vi "CryoCooler Alarm Check.vi"(8 "error in (no error)":errorcluster, 10 "Cryo Alarms":T1, 11 "Array":T3[](array[typedef])) -> (0 "error out":errorcluster, 1 "shutdown?":bool, 2 "Alarms":T2[](array[typedef]), 3 "Alarm":bool)   [LabVIEW 2024]
uses:
  Cryo Cooler/CryoCoolerAVC/CryoCoolerAVC Status Cluster.ctl
  typedefs/CC cluster Alarm Data.ctl
  CryoCooler cluster Alarm Settings.ctl
  Cryo Cooler/CryoCoolerAVC/CryoCoolerAVC.lvclass
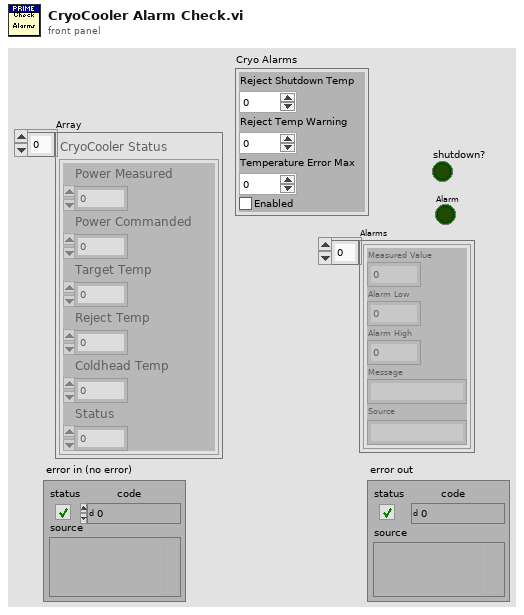
[diagram p1: front panel]
types:
  T1 = typedef "CryoCooler cluster Alarm Settings.ctl" = cluster{"Reject Shutdown Temp":dbl, "Reject Temp Warning":dbl, "Temperature Error Max":dbl, "Enabled":bool}
  T2 = typedef "CC cluster Alarm Data.ctl" = cluster{"Measured Value":dbl, "Alarm Low":dbl, "Alarm High":dbl, "Message":string, "Source":string}
  T3 = typedef "CryoCoolerAVC.lvclass/CryoCoolerAVC Status Cluster.ctl" = cluster{"Power Measured":dbl, "Power Commanded":dbl, "Target Temp":dbl, "Reject Temp":dbl, "Coldhead Temp":dbl, "Status":dbl}
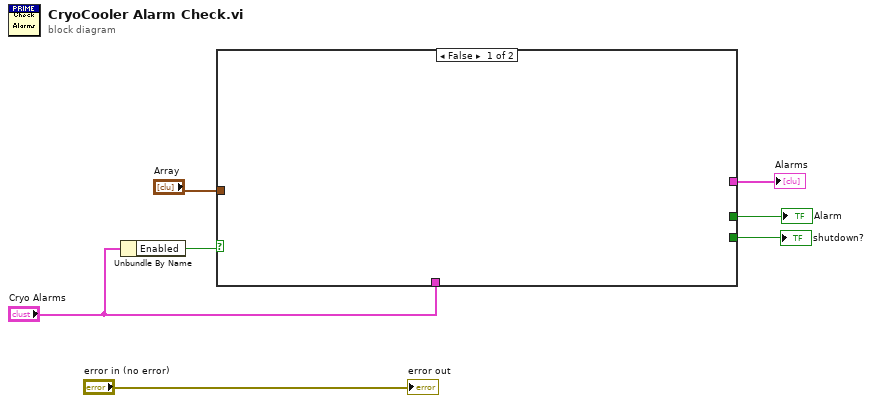
[diagram p0: block diagram]
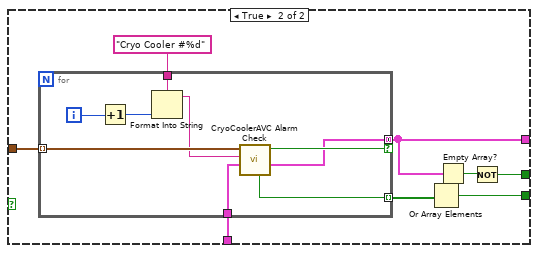
[diagram p2: hidden frame]
diagram:
  n1 = Unbundle By Name("Cryo Alarms") -> ("Enabled"=w1:bool)
  n2 = case shown="False" w1 {
    tunnel: "Array" -> [_ w14]
    tunnel: [_ w13] -> w5
    tunnel: [_ w11] -> w4
    tunnel: [_ w9] -> w3
    tunnel: "Cryo Alarms" -> [_ w8]
    frame False {
    }
    frame True {
      n3 = for {
        tunnel: w14 -> [w24] mode=indexing
        tunnel: "Cryo Cooler #%d" ("format string") -> [w23]
        tunnel: [w19] -> w13 mode=concatenating if=w20
        tunnel: w8 -> [w17]
        tunnel: [w16] -> w10 mode=indexing
        i -> [w22]
        n4 = Increment(x=w22) -> (x+1=w21:i32)
        n5 = Format Into String(format string=w23, w21) -> (resulting string=w18:string)  [unwired: 2 in, 1 out]
        n6 = call "CryoCoolerAVC Alarm Check.vi"("Cryo Alarms"=w17, "Cryocooler"=w18, "CryoCooler Status"=w24) -> ("Alarms"=w19:T2[], "alarm"=w20:bool, "Shutdown?"=w16:bool)  [unwired: 4 in, 2 out]
      }
      n7 = Or Array Elements(Boolean array=w10) -> (logical OR=w9:bool)
      n8 = Empty Array?(array=w13) -> (empty?=w12:bool)
      n9 = Not(x=w12) -> (.not. x?=w11:bool)
    }
  }
  "Alarm" <- w4
  "Alarms" <- w5
  "shutdown?" <- w3
  "error out" <- "error in (no error)"
